vi "MT_read_failed.vi"(8 "error in":errorcluster, 9 "sampling rate":dbl) -> (0 "error out":errorcluster, 2 "data":waveform(dbl)[](array[waveform]))   [LabVIEW 2019]
uses:
  <vilib>/DAQmx/read.llb/DAQmx Read (Analog 1D Wfm NChan NSamp).vi
  <vilib>/DAQmx/create/channels.llb/DAQmx Create Channel (AI-Voltage-Basic).vi
  <vilib>/DAQmx/configure/timing.llb/DAQmx Timing (Sample Clock).vi
  <vilib>/DAQmx/miscellaneous.llb/DAQmx Fill In Error Info.vi
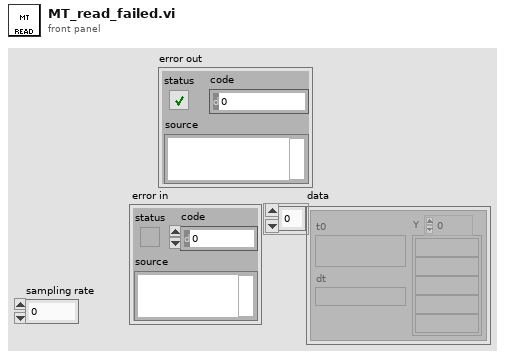
[diagram p1: front panel]
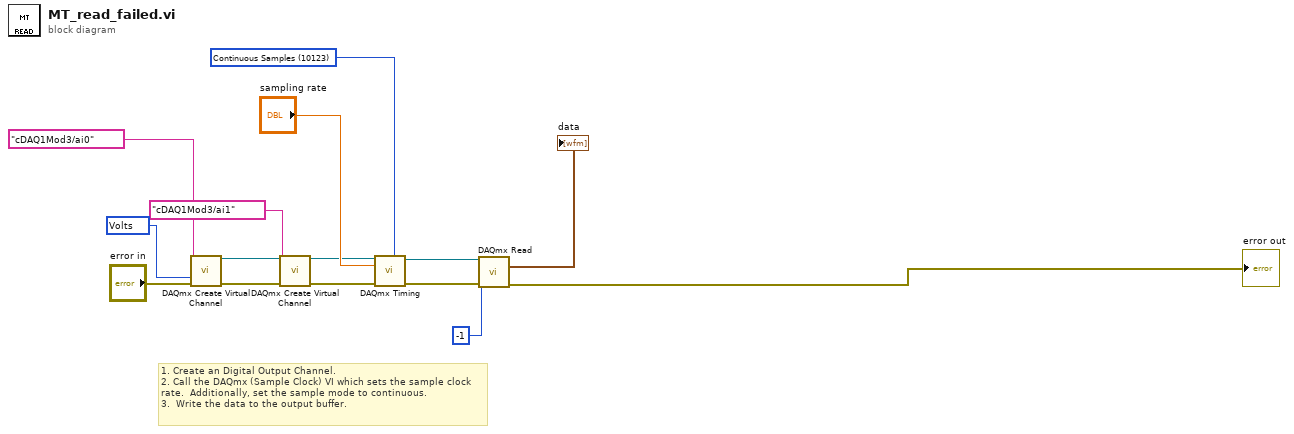
[diagram p0: block diagram]
diagram:
  w12 = 10348 items=["Volts"=10348, "From Custom Scale"=10065] ("units")
  w14 = 10123 items=["Finite Samples"=10178, "Continuous Samples"=10123] ("sample mode")
  # "1. Create an Digital Output Channel. \n2. Call the DAQmx (Sample Clock) VI which sets the sample clock rate.  Additionally, set the sample mode to continuous.\n3.  Write the data to the output buffer."
  n1 = call-poly <vilib>:"DAQmx Create Virtual Channel.vi"("physical channels"=tag "cDAQ1Mod3/ai0", "units"=w12, "error in"="error in") -> ("task out"=w11:refnum<k21>, "error out"=w10:errorcluster)  [unwired: 6 in, 5 out]
  n2 = call-poly <vilib>:"DAQmx Create Virtual Channel.vi"("task in"=w11, "physical channels"=tag "cDAQ1Mod3/ai1", "error in"=w10) -> ("task out"=w9:refnum<k21>, "error out"=w8:errorcluster)  [unwired: 11 in]
  n3 = call-poly <vilib>:"DAQmx Timing.vi"("task/channels in"=w9, "sample mode"=w14, "rate"="sampling rate", "error in"=w8) -> ("task out"=w5:refnum<k21>, "error out"=w4:errorcluster)  [unwired: 3 in, 7 out]
  n4 = call-poly <vilib>:"DAQmx Read.vi"("task/channels in"=w5, "number of samples per channel"=-1, "error in"=w4) -> ("data"=→"data":waveform(dbl)[], "error out"=→"error out":errorcluster)  [unwired: 10 in, 1 out]
